vi "IMAQ-GetContrast.vi"(5 "Image Device IN":cluster{"Image":T1, "errorImage":errorcluster}) -> (1 "Contraste":dbl format="%.2f", 2 "Image Device OUT":cluster{"Image":T1, "errorImage":errorcluster})   [LabVIEW 2010]
uses:
  <vilib>/vision/Image Controls.llb/IMAQ Image.ctl
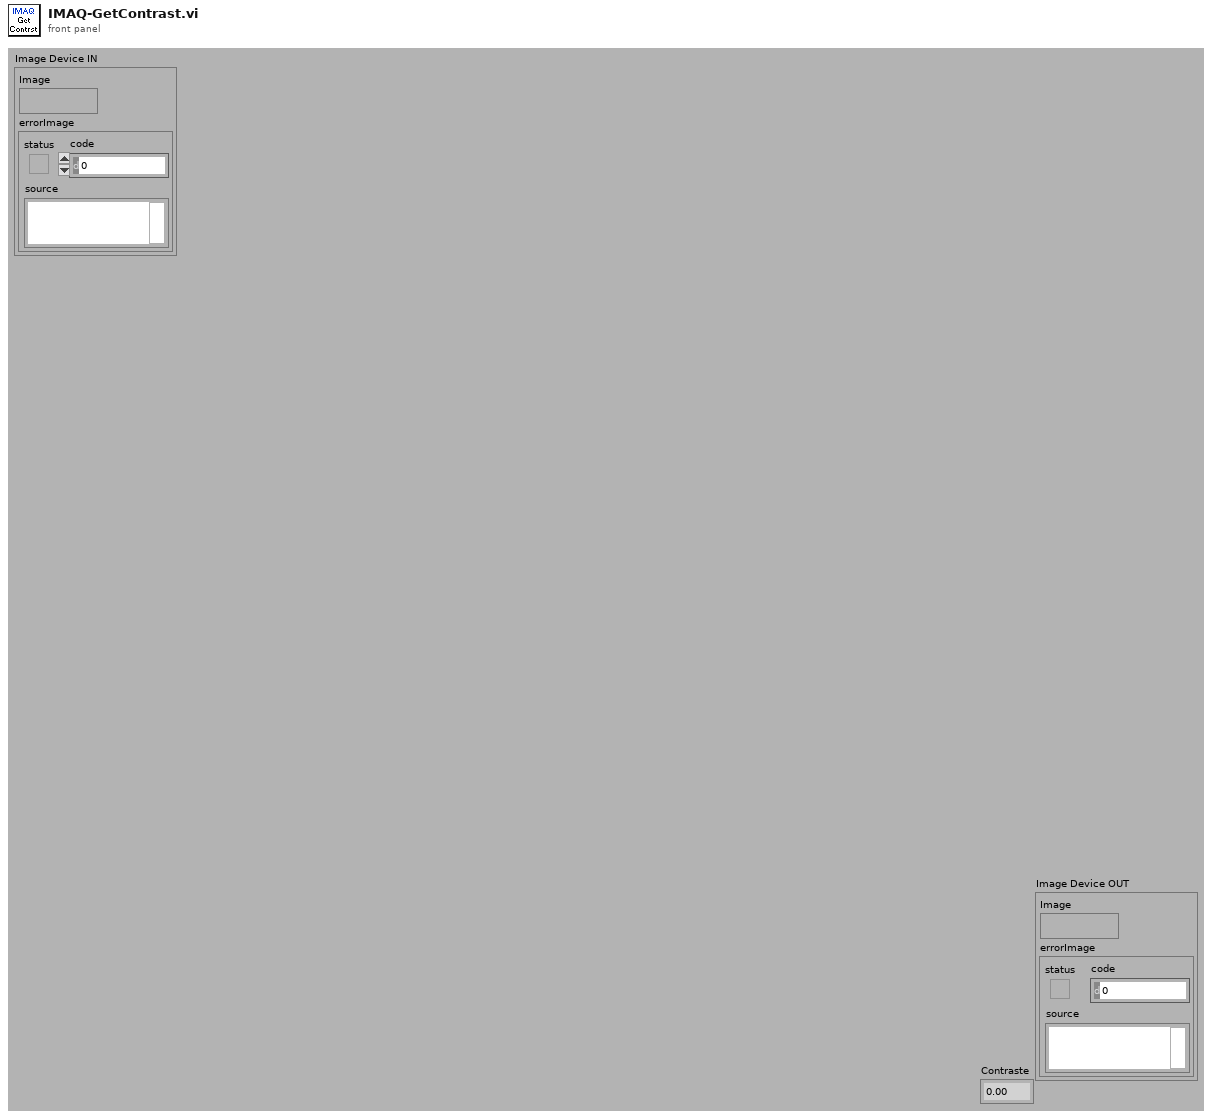
[diagram p1: front panel]
types:
  T1 = typedef "IMAQ Image.ctl" = refnum<image>
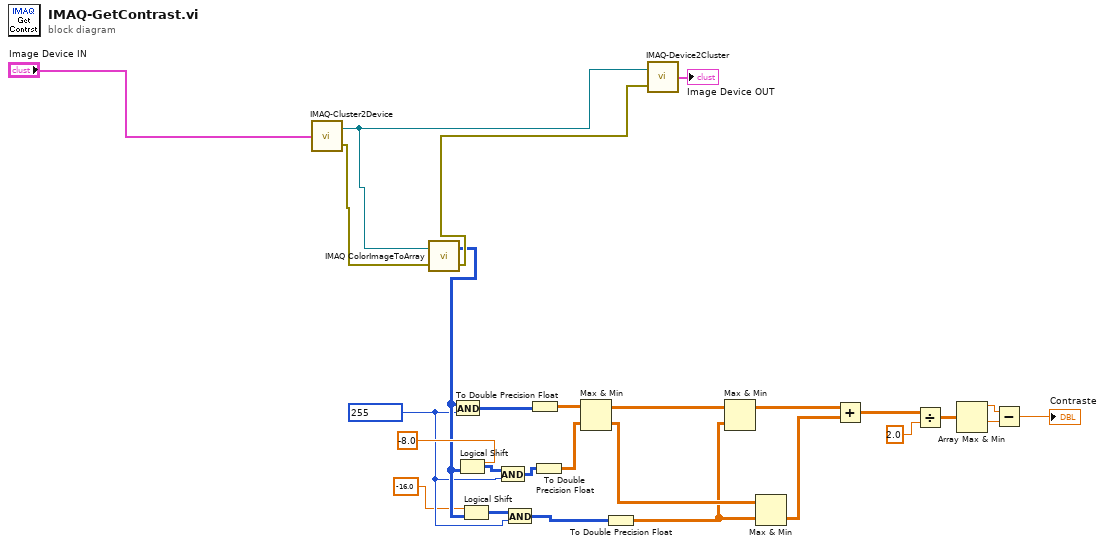
[diagram p0: block diagram]
diagram:
  w4 = u32 255
  n1 = call "IMAQ-Cluster2Device.vi"("Image Device IN"="Image Device IN") -> ("errorImage OUT"=w24:errorcluster, "Image OUT"=w25:T1)
  n2 = call "IMAQ ColorImageToArray"("Image"=w25, "error in (no error)"=w24) -> ("Image Pixels (U32)"=w7:u32[][], "error out"=w23:errorcluster)  [unwired: 2 in, 1 out]
  n3 = And(x=w7, y=w4) -> (x .and. y?=w11:u32[][])
  n4 = Logical Shift(y=sgl -8.0 ("x"), x=w7) -> (x << y=w6:u32[][])
  n5 = Logical Shift(y=sgl -16.0 ("x"), x=w7) -> (x << y=w5:u32[][])
  n6 = And(x=w6, y=w4) -> (x .and. y?=w3:u32[][])
  n7 = And(x=w5, y=w4) -> (x .and. y?=w2:u32[][])
  n8 = To Double Precision Float(number=w11) -> (double precision float=w12:dbl[][])
  n9 = To Double Precision Float(number=w3) -> (double precision float=w10:dbl[][])
  n10 = Max & Min(x=w12, y=w10) -> (max(x,y)=w22:dbl[][], min(x,y)=w21:dbl[][])
  n11 = To Double Precision Float(number=w2) -> (double precision float=w9:dbl[][])
  n12 = call "IMAQ-Device2Cluster.vi"("errorImage IN"=w23, "Image IN"=w25) -> ("Image Device OUT"=→"Image Device OUT":cluster{"Image":T1, "errorImage":errorcluster})
  n13 = Max & Min(x=w22, y=w9) -> (max(x,y)=w19:dbl[][])  [unwired: 1 out]
  n14 = Max & Min(x=w21, y=w9) -> (min(x,y)=w18:dbl[][])  [unwired: 1 out]
  n15 = Add(x=w19, y=w18) -> (x+y=w17:dbl[][])
  n16 = Divide(x=w17, y=2.0) -> (x/y=w14:dbl[][])
  n17 = Array Max & Min(array=w14) -> (max value=w15:dbl, min value=w16:dbl)  [unwired: 2 out]
  n18 = Subtract(x=w15, y=w16) -> (x-y=→"Contraste":dbl)
